vi "Up_CalibCircle.vi"(0 "ImageIn":T4, 5 "Data":T1, 9 "Lower value":sgl, 11 "error in":errorcluster) -> (4 "Image Out":T4(plugin-control), 6 "CyclePosition":cluster{"X":sgl, "Y":sgl}, 8 "Pass":bool, 10 "Radius":dbl, 15 "error out":errorcluster)   [LabVIEW 2019]
uses:
  <vilib>/vision/Image Controls.llb/IMAQ Image.ctl
  <vilib>/vision/NI_Vision_Development_Module.lvlib
panel:
  out "size(s)":i32
  out "Circles":T2(array[cluster])
  out "Circles Data (calibrated)":T3(array[cluster])
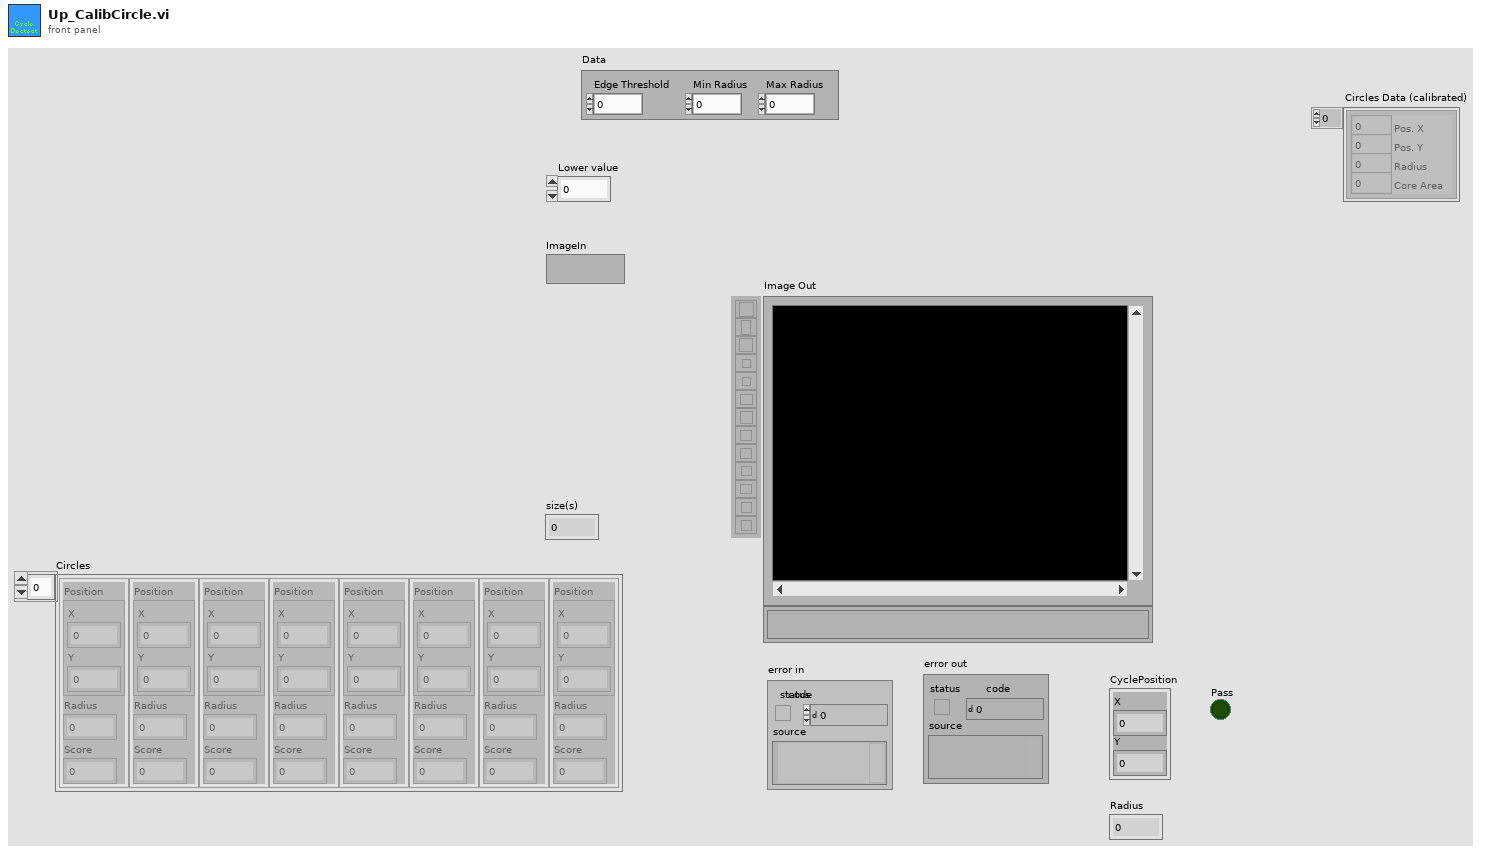
[diagram p1: front panel]
types:
  T1 = cluster{"Edge Threshold":i32, "Min Radius":dbl, "Max Radius":dbl}
  T2 = cluster{"Position":cluster{"X":sgl, "Y":sgl}, "Radius":dbl, "Score":dbl}[]
  T3 = cluster{"Pos. X":i32, "Pos. Y":i32, "Radius":i32, "Core Area":i32}[]
  T4 = typedef "IMAQ Image.ctl" = refnum<image>
  T5 = enum32{"Linear", "Log", "Exp", "Square", "Square root", "Power X", "Power 1/X"}
  T6 = typedef "Image Type" = u32
  T7 = cluster{"histogram":u32[], "Minimal Value":sgl, "Maximal Value":sgl, "Starting Value":sgl, "Interval Width":sgl, "Mean Value":sgl, "Standard  Variation":sgl, "Area (pixels)":i32}
  T8 = cluster{"Rotation":bool, "Scale":bool, "Occlusion":bool, "Range Settings":cluster{"Match Constraints":u32, "Min":dbl, "Max":dbl}[]}
  T9 = cluster{"Extraction Mode":u32, "Edge Threshold":i32, "Edge Filter Size":u32, "Min Length":i32, "Row Search Step Size":i32, "Col Search Step Size":i32, "Max Endpoint Gap":i32, "Closed":bool, "Subpixel":bool}
  T10 = cluster{"Global Rectangle":i32[], "Contours":cluster{"ID":enum32{"External", "Internal"}, "Type":u32, "Coordinates":i32[]}[]}
  T11 = cluster{"Position":cluster{"X":sgl, "Y":sgl}, "Radius":dbl, "Score":dbl}
  T12 = cluster{"Pos. X":i32, "Pos. Y":i32, "Radius":i32, "Core Area":i32}
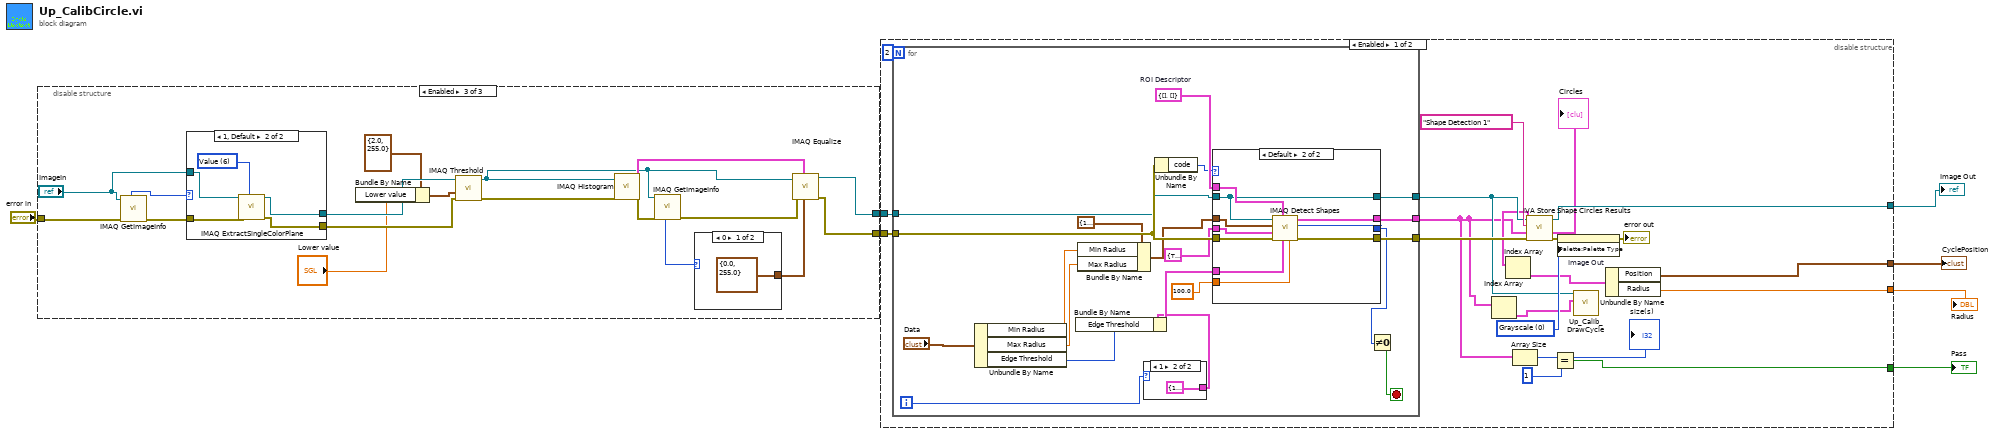
[diagram p0: block diagram]
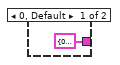
[diagram p2: hidden frame]
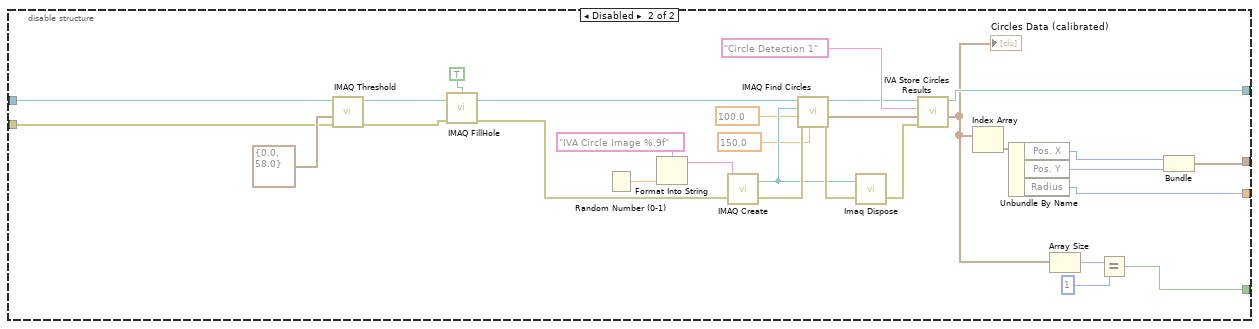
[diagram p4: hidden frame]
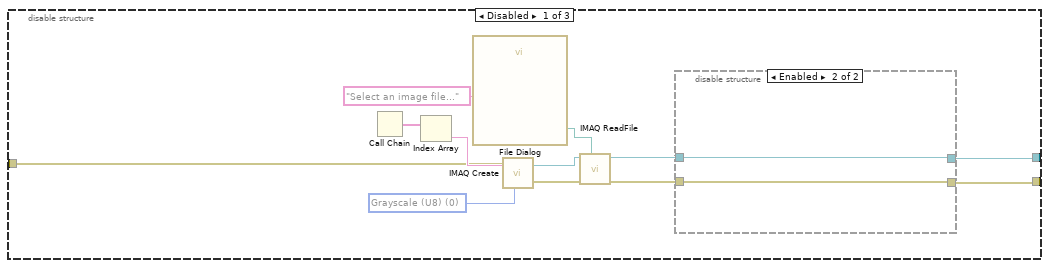
[diagram p5: hidden frame]
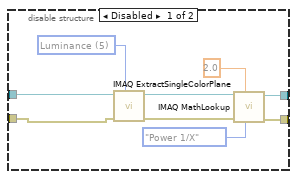
[diagram p6: hidden frame]
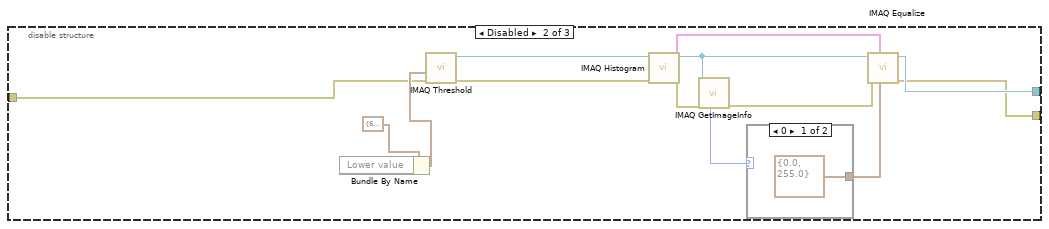
[diagram p7: hidden frame]
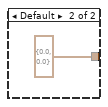
[diagram p8: hidden frame]
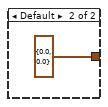
[diagram p9: hidden frame]
diagram:
  n1 = disable-structure shown="Enabled" {
    disable-tunnel: [w10 w32 w55] -> w7
    disable-tunnel: [w9 w36 w54] -> w6
    disable-tunnel: "error in" -> [w8 w31 w62]
    frame Disabled {
      w13 = T6 0 items=["Grayscale (U8)", "Grayscale (I16)", "Grayscale (SGL)", "Complex (CSG)", "RGB (U32)", "HSL (U32)", "RGB (U64)", "Grayscale (U16)"] ("Image Type")
      n2 = Call Chain() -> (call chain=w17:string[])
      n3 = Index Array(array=w17) -> (element=w16:string)  [unwired: 1 in]
      n4 = call "File Dialog"("prompt"="Select an image file...") -> ("selected path"=w14:path)  [unwired: 6 in, 8 out]
      n5 = call "IMAQ Create"("Image Name"=w16, "Image Type"=w13, "error in (no error)"=w8) -> ("New Image"=w19:T4, "error out"=w18:errorcluster)  [unwired: 1 in, 1 out]
      n6 = call "IMAQ ReadFile"("File Path"=w14, "error in (no error)"=w18, "Image"=w19) -> ("error out"=w11:errorcluster, "Image Out"=w12:T4)  [unwired: 2 in, 5 out]
      n7 = disable-structure shown="Enabled" {
        disable-tunnel: w12 -> [w27 w30]
        disable-tunnel: w11 -> [w26 w29]
        disable-tunnel: [w21 w29] -> w10
        disable-tunnel: [w20 w30] -> w9
        frame Disabled {
          w28 = 5 items=["Red", "Green", "Blue", "Hue", "Saturation", "Luminance", "Value", "Intensity"] ("Color Plane")
          n8 = call "IMAQ ExtractSingleColorPlane"("Color Plane"=w28, "error in (no error)"=w26, "Image Src"=w27) -> ("error out"=w22:errorcluster, "Image Dst Out"=w23:T4)  [unwired: 7 in]
          n9 = call "IMAQ MathLookup"("Operator"=T5."Power 1/X", "X Value"=sgl 2.0, "error in (no error)"=w22, "Image Src"=w23) -> ("error out"=w21:errorcluster, "Image Dst Out"=w20:T4)  [unwired: 6 in]
        }
        frame Enabled {
        }
      }
    }
    frame Disabled {
      n10 = Bundle By Name(cluster=cluster{"Lower value":sgl, "Upper value":sgl} {"Lower value"=60.0, "Upper value"=255.0} ("Range")) -> (w34:cluster{"Lower value":sgl, "Upper value":sgl}, "Lower value"=w33:sgl)
      n11 = call "IMAQ Threshold"("error in (no error)"=w31, "Range"=w34) -> ("error out"=w44:errorcluster, "Image Dst Out"=w41:T4, "Image Src"=w37:T4)  [unwired: 3 in, 4 out]
      n12 = call "IMAQ Histogram"("error in (no error)"=w44, "Image"=w41) -> ("error out"=w40:errorcluster, "Histogram Report"=w43:T7)  [unwired: 3 in, 5 out]
      n13 = call "IMAQ GetImageInfo"("error in (no error)"=w40, "Image"=w41) -> ("error out"=w39:errorcluster, "Image Type"=w42:T6)  [unwired: 8 out]
      n14 = case shown="0" w42 {
        tunnel: [cluster{"Minimum":sgl, "Maximum":sgl} {"Minimum"=0.0, "Maximum"=255.0} ("Range") cluster{"Minimum":sgl, "Maximum":sgl} {"Minimum"=0.0, "Maximum"=0.0} ("Range")] -> w38
        frame 0 {
        }
        frame Default {
        }
      }
      n15 = call "IMAQ Equalize"("Range"=w38, "Histogram Report"=w43, "error in (no error)"=w39, "Image Src"=w41) -> ("error out"=w32:errorcluster, "Image Dst Out"=w36:T4)  [unwired: 2 in, 4 out]
    }
    frame Enabled {
      n16 = call "IMAQ GetImageInfo"("error in (no error)"=w62, "Image"="ImageIn") -> ("error out"=w61:errorcluster, "Image Type"=w64:T6)  [unwired: 2 in, 6 out]
      n17 = case shown="1, Default" w64 {
        tunnel: [w68 w72] -> w51
        tunnel: "ImageIn" -> [w68 w71]
        tunnel: w61 -> [w67 w70]
        tunnel: [w67 w69] -> w50
        frame 0 {
        }
        frame 1, Default {
          w73 = 6 items=["Red", "Green", "Blue", "Hue", "Saturation", "Luminance", "Value", "Intensity"] ("Color Plane")
          n18 = call "IMAQ ExtractSingleColorPlane"("Color Plane"=w73, "error in (no error)"=w70, "Image Src"=w71) -> ("error out"=w69:errorcluster, "Image Dst Out"=w72:T4)  [unwired: 7 in]
        }
      }
      n19 = Bundle By Name(cluster=cluster{"Lower value":sgl, "Upper value":sgl} {"Lower value"=2.0, "Upper value"=255.0} ("Range"), "Lower value"="Lower value") -> (w48:cluster{"Lower value":sgl, "Upper value":sgl})
      n20 = call "IMAQ Threshold"("error in (no error)"=w50, "Range"=w48, "Image Src"=w51) -> ("error out"=w52:errorcluster, "Image Dst Out"=w53:T4)  [unwired: 7 in]
      n21 = call "IMAQ Histogram"("error in (no error)"=w52, "Image"=w53) -> ("error out"=w58:errorcluster, "Histogram Report"=w56:T7)  [unwired: 3 in, 5 out]
      n22 = call "IMAQ GetImageInfo"("error in (no error)"=w58, "Image"=w53) -> ("error out"=w59:errorcluster, "Image Type"=w57:T6)  [unwired: 8 out]
      n23 = case shown="0" w57 {
        tunnel: [cluster{"Minimum":sgl, "Maximum":sgl} {"Minimum"=0.0, "Maximum"=255.0} ("Range") cluster{"Minimum":sgl, "Maximum":sgl} {"Minimum"=0.0, "Maximum"=0.0} ("Range")] -> w60
        frame 0 {
        }
        frame Default {
        }
      }
      n24 = call "IMAQ Equalize"("Range"=w60, "Histogram Report"=w56, "error in (no error)"=w59, "Image Src"=w53) -> ("error out"=w55:errorcluster, "Image Dst Out"=w54:T4)  [unwired: 2 in, 4 out]
    }
  }
  n25 = disable-structure shown="Enabled" {
    disable-tunnel: w7 -> [w92 w136]
    disable-tunnel: w6 -> [w91 w137]
    disable-tunnel: [w85 w132] -> w5
    disable-tunnel: [w80 w135] -> w4
    disable-tunnel: [w79 w131] -> w3
    disable-tunnel: [w78 w126] -> w2
    frame Enabled {
      w87 = u32 0 items=["Grayscale", "Binary", "Gradient", "Rainbow", "Temperature", "User Defined"] ("Palette")
      n26 = for {
        N: 2 -> [_]
        tunnel: w92 -> [w112]
        tunnel: w91 -> [w108]
        tunnel: [w107] -> w90
        tunnel: [w105] -> w84
        tunnel: [w97] -> w76
        i -> [w96]
        stop <- w93 stop-if-true
        w109 = T10 {"Global Rectangle"=[], "Contours"=[]}  # ROI Descriptor
        n27 = Unbundle By Name("Data") -> ("Min Radius"=w100:dbl, "Max Radius"=w99:dbl, "Edge Threshold"=w101:i32)
        n28 = Bundle By Name(cluster=cluster{"Min Radius":dbl, "Max Radius":dbl} {"Min Radius"=110.0, "Max Radius"=140.0} ("Circle Descriptor"), "Min Radius"=w100, "Max Radius"=w99) -> (w104:cluster{"Min Radius":dbl, "Max Radius":dbl})
        n29 = case shown="1" w96 {
          tunnel: [T9 {"Extraction Mode"=0, "Edge Threshold"=90, "Edge Filter Size"=1, "Min Length"=25, "Row Search Step Size"=15, "Col Search Step Size"=15, "Max Endpoint Gap"=10, "Closed"=FALSE, "Subpixel"=FALSE} ("Curve Parameters") T9 {"Extraction Mode"=1, "Edge Threshold"=90, "Edge Filter Size"=1, "Min Length"=25, "Row Search Step Size"=15, "Col Search Step Size"=15, "Max Endpoint Gap"=10, "Closed"=FALSE, "Subpixel"=FALSE} ("Curve Parameters")] -> w95
          frame 0, Default {
          }
          frame 1 {
          }
        }
        n30 = Bundle By Name(cluster=w95, "Edge Threshold"=w101) -> (w102:T9)
        n31 = Unbundle By Name(w112) -> ("code"=w106:i32)
        n32 = case shown="Default" w106 {
          tunnel: w112 -> [_ w125]
          tunnel: [_ w124] -> w94
          tunnel: T8 {"Rotation"=TRUE, "Scale"=FALSE, "Occlusion"=FALSE, "Range Settings"=[{"Match Constraints"=0, "Min"=0.0, "Max"=360.0}]} ("Match Options") -> [_ w123]
          tunnel: w102 -> [_ w122]
          tunnel: 100.0 ("Minimum match score") -> [_ w121]
          tunnel: w104 -> [_ w120]
          tunnel: w109 -> [_ w119]
          tunnel: [_ w118] -> w97
          tunnel: w108 -> [w115 w116]
          tunnel: [_ w117] -> w107
          tunnel: [w115 w116] -> w105
          frame -1074396199, -1074396198 {
            # "Discard Coordinate\nSystem Error"
          }
          frame Default {
            n33 = call-poly "IMAQ Detect Shapes"("Minimum match score"=w121, "Curve Parameters"=w122, "ROI Descriptor"=w119, "error in (no error)"=w125, "Match Options"=w123, "Circle Descriptor"=w120, "Image"=w116) -> ("error out"=w117:errorcluster, "Number of Matches Returned"=w124:i32, "Circles"=w118:T2)  [unwired: 2 in]
          }
        }
        n34 = Not Equal To 0?(x=w94) -> (x != 0?=w93:bool)
      }
      n35 = Index Array(array=w76) -> (element=w75:T11)  [unwired: 1 in]
      n36 = Array Size(array=w76) -> (size(s)=w82:i32)
      "size(s)" <- w82
      n37 = call <vilib>:"IVA Store Shape Circles Results.vi"("error in (no error)"=w90, "Circles"=w76, "Step Name"="Shape Detection 1", "Image in"=w84) -> ("error out"=w89:errorcluster, "Circles (Calibrated)"=w77:T2, "Image dup"=w79:T4)  [unwired: 5 in]
      "Circles" <- w77
      n38 = Index Array(array=w77) -> (element=w83:T11)  [unwired: 1 in]
      n39 = Equal?(x=w82, y=1) -> (x = y?=w78:bool)
      n40 = property on="Image Out" class="ImageControl"(error in=w89, "Palette:Palette Type"=w87) -> (error out=→"error out":errorcluster)  [unwired: 1 in, 1 out]
      n41 = call "Up_Calib_DrawCycle.vi"("CirclesDataIn"=w75, "ImageIn"=w84) -> ()  [unwired: 9 in, 1 out]
      n42 = Unbundle By Name(w83) -> ("Position"=w85:cluster{"X":sgl, "Y":sgl}, "Radius"=w80:dbl)
    }
    frame Disabled {
      n43 = call "IMAQ Threshold"("error in (no error)"=w136, "Range"=cluster{"Lower value":sgl, "Upper value":sgl} {"Lower value"=0.0, "Upper value"=58.0}, "Image Src"=w137) -> ("error out"=w139:errorcluster, "Image Dst Out"=w141:T4)  [unwired: 3 in, 4 out]
      n44 = call "IMAQ FillHole"("error in (no error)"=w139, "Image Src"=w141, "Connectivity 4/8 (8)"=TRUE) -> ("error out"=w142:errorcluster, "Image Dst Out"=w149:T4)  [unwired: 1 in, 2 out]
      n45 = Random Number (0-1)() -> (number: 0 to 1=w153:dbl)
      n46 = Format Into String(format string="IVA Circle Image %.9f" ("Image Name"), w153) -> (resulting string=w151:string)  [unwired: 2 in, 1 out]
      n47 = call "IMAQ Create"("Image Name"=w151, "error in (no error)"=w142) -> ("New Image"=w145:T4, "error out"=w146:errorcluster)  [unwired: 2 in, 1 out]
      n48 = call "IMAQ Find Circles"("Max Radius"=sgl 150.0, "error in (no error)"=w146, "Min Radius"=sgl 100.0, "Image Dst"=w145, "Image Src"=w149) -> ("error out"=w147:errorcluster, "Circles Data"=w130:T3)  [unwired: 5 out]
      n49 = call "Imaq Dispose"("Image"=w145, "error in (no error)"=w147) -> ("error out"=w148:errorcluster)  [unwired: 1 in, 3 out]
      n50 = call <vilib>:"IVA Store Circles Results.vi"("error in (no error)"=w148, "Circles Data"=w130, "Step Name"="Circle Detection 1", "Image in"=w149) -> ("Circles Data (calibrated)"=w127:T3, "Image dup"=w131:T4)  [unwired: 6 out]
      "Circles Data (calibrated)" <- w127
      n51 = Index Array(array=w127) -> (element=w154:T12)  [unwired: 1 in]
      n52 = Unbundle By Name(w154) -> ("Pos. X"=w134:i32, "Pos. Y"=w133:i32, "Radius"=w135:i32)
      n53 = Array Size(array=w127) -> (size(s)=w129:i32)
      n54 = Equal?(x=w129, y=1) -> (x = y?=w126:bool)
      n55 = Bundle("Pos. X"=w134, "Pos. Y"=w133) -> (w132:cluster{"Pos. X":i32, "Pos. Y":i32})  [unwired: 1 in]
    }
  }
  "CyclePosition" <- w5
  "Radius" <- w4
  "Image Out" <- w3
  "Pass" <- w2
